vi "HEWH Dip Tube Pressure Compensation.vi"(11 "GPM Target":dbl) -> (3 "Updated Flow Rate (GPM)":dbl)   [LabVIEW 2023]
panel:
  out "y":dbl
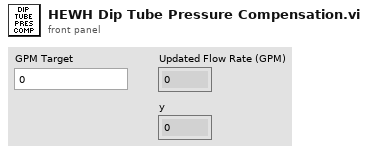
[diagram p1: front panel]
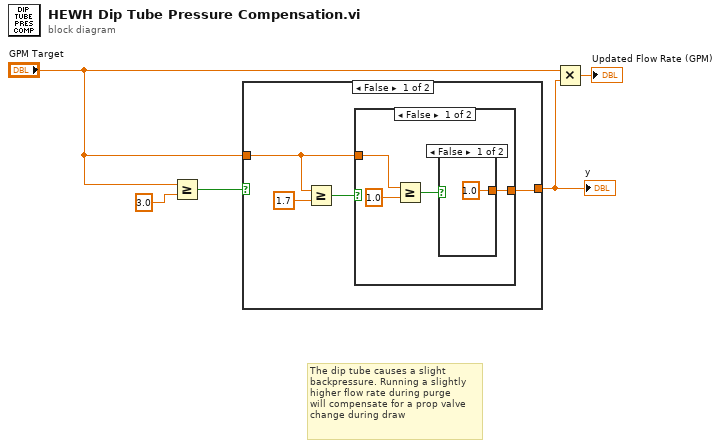
[diagram p0: block diagram]
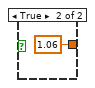
[diagram p2: hidden frame]
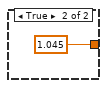
[diagram p3: hidden frame]
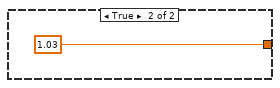
[diagram p4: hidden frame]
diagram:
  # "The dip tube causes a slight\nbackpressure. Running a slightly\nhigher flow rate during purge\nwill compensate for a prop valve\nchange during draw"
  n1 = Greater Or Equal?(x="GPM Target", y=3.0) -> (x >= y?=w2:bool)
  n2 = case shown="False" w2 {
    tunnel: [w7 1.03 ("y")] -> w4
    tunnel: "GPM Target" -> [w6 _]
    frame False {
      n3 = Greater Or Equal?(x=w6, y=1.7) -> (x >= y?=w8:bool)
      n4 = case shown="False" w8 {
        tunnel: [w13 1.045 ("y")] -> w7
        tunnel: w6 -> [w12 _]
        frame False {
          n5 = Greater Or Equal?(x=w12, y=1.0) -> (x >= y?=w10:bool)
          n6 = case shown="False" w10 {
            tunnel: [1.0 ("y") 1.06 ("y")] -> w13
            frame False {
            }
            frame True {
            }
          }
        }
        frame True {
        }
      }
    }
    frame True {
    }
  }
  "y" <- w4
  n7 = Multiply(x="GPM Target", y=w4) -> (x*y=→"Updated Flow Rate (GPM)":dbl)
